vi "GtoDegree.vi"(11 "PathPointG":cluster{dbl, i32}) -> (3 "steer":dbl)   [LabVIEW 2015]
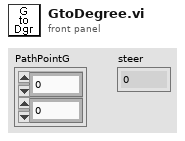
[diagram p1: front panel]
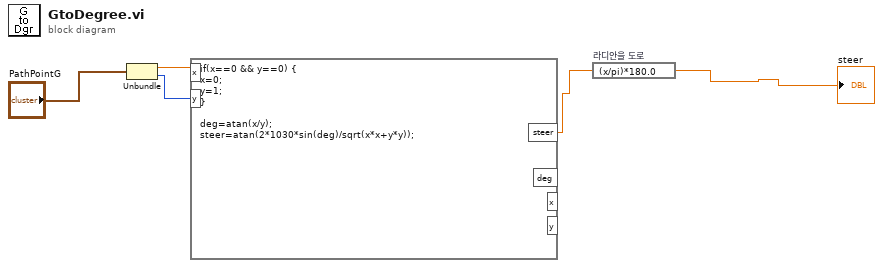
[diagram p0: block diagram]
diagram:
  n1 = Unbundle("PathPointG") -> (w1:dbl, w2:i32)
  n2 = formula code="if(x==0 && y==0) {\nx=0;\ny=1;\n}\n\ndeg=atan(x/y);\nsteer=atan(2*1030*sin(deg)/sqrt(x*x+y*y));"("x"=w1, "y"=w2) -> ("steer"=w3:dbl)  [unwired: 3 out]
  n3 = expression code="(x/pi)*180.0" "라디안을 도로"(w3) -> (→"steer":dbl)
